vi "StanleyMethod.vi"(0 "¥÷(Heading Err)radian":dbl, 1 "e(Cross-Track Err)m/s":dbl, 2 "kappa":dbl format="%#_13g", 3 "v(Velocity)m/s":dbl, 4 "k(Gain)":dbl) -> (5 "ヤ(OutputSteer)degrees":dbl, 6 "ヤ(OutputSteer)radian":dbl)   [LabVIEW 2024]
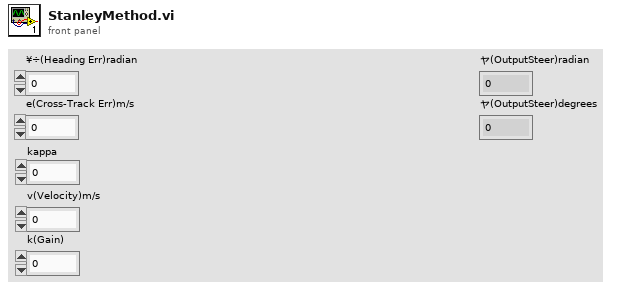
[diagram p1: front panel]
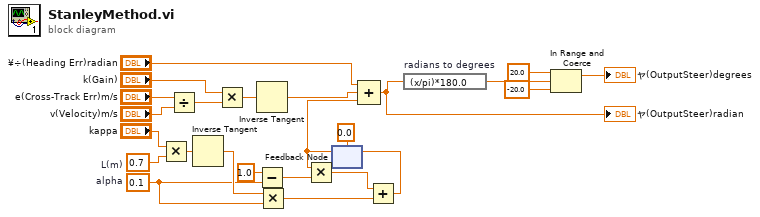
[diagram p0: block diagram]
diagram:
  w8 = 0.1  # alpha
  w14 = 0.7  # L(m)
  n1 = Multiply(x="kappa", y=w14) -> (x*y=w13:dbl)
  n2 = Divide(x="e(Cross-Track Err)m/s", y="v(Velocity)m/s") -> (x/y=w23:dbl)
  n3 = Inverse Tangent(1:w13) -> (0:w9:dbl)
  n4 = Multiply(x="k(Gain)", y=w23) -> (x*y=w24:dbl)
  n5 = Inverse Tangent(1:w24) -> (0:w3:dbl)
  n6 = Subtract(x=1.0, y=w8) -> (x-y=w5:dbl)
  n7 = Multiply(x=w9, y=w8) -> (x*y=w6:dbl)
  n8 = feedback #1(0.0) -> (w4:dbl)
  n9 = Multiply(x=w4, y=w5) -> (x*y=w7:dbl)
  n10 = Compound Arithmetic op=ADD("¥÷(Heading Err)radian", w3, w4) -> (w1:dbl)
  "ヤ(OutputSteer)radian" <- w1
  n11 = Add(x=w7, y=w6) -> (x+y=w11:dbl)
  n12 = feedback-in #1(w11) -> ()
  n13 = expression code="(x/pi)*180.0" "radians to degrees"(w1) -> (w16:dbl)
  n14 = In Range and Coerce(upper limit=20.0, x=w16, lower limit=-20.0) -> (coerced(x)=→"ヤ(OutputSteer)degrees":dbl)  [unwired: 1 out]
